vi "Channel Array Size Error Test.vi"(8 "error in":errorcluster, 11 "NI 9227 test in":refnum<class "NI 9227 Test.lvclass">) -> (0 "error out":errorcluster, 3 "NI 9227 test out":refnum<class "NI 9227 Test.lvclass">)   [LabVIEW 2019, in "NI 9227 Test.lvclass"]
uses:
  NI 9227 Test.lvclass
  Module Test.lvclass
  Scripting/Modules/NI 9227/NI 9227.lvclass
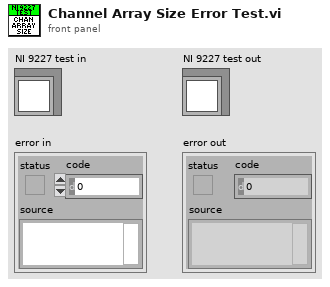
[diagram p1: front panel]
types:
  T1 = typedef "Scan Engine Scripting.lvlib/analog channel settings.ctl" = cluster{"name":string, "default value":dbl}
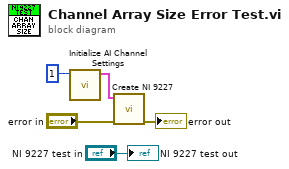
[diagram p0: block diagram]
diagram:
  n1 = call "Initialize AI Channel Settings.vi"("array size"=1) -> ("channel settings"=w4:T1[])  [unwired: 10 in]
  n2 = call "Create NI 9227.vi"("error in"="error in", "channel settings"=w4) -> ("error out"=→"error out":errorcluster)  [unwired: 8 in, 1 out]
  "NI 9227 test out" <- "NI 9227 test in"
